vi "Read Wait For Response.vi"(0 "LVx.lvclass in":refnum<class "LVx.lvclass">, 11 "error in (no error)":errorcluster) -> (4 "LVx.lvclass out":refnum<class "LVx.lvclass">, 6 "Wait For Response?":bool, 15 "error out":errorcluster)   [LabVIEW 2011, in "LVx.lvlib" / "LVx.lvclass"]
uses:
  LVx.lvclass
  LVx.lvclass/LVx.ctl
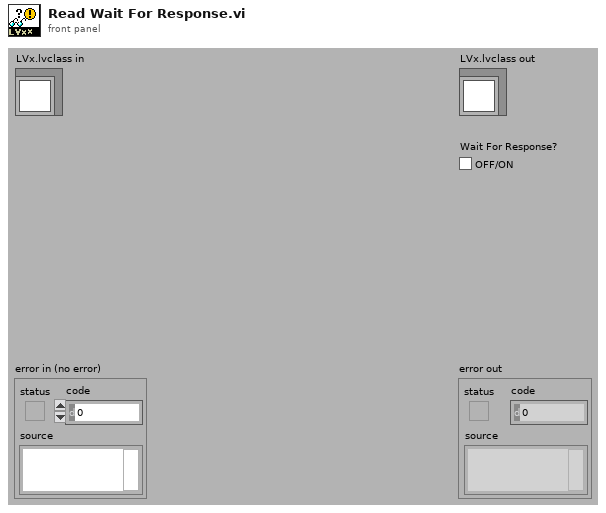
[diagram p1: front panel]
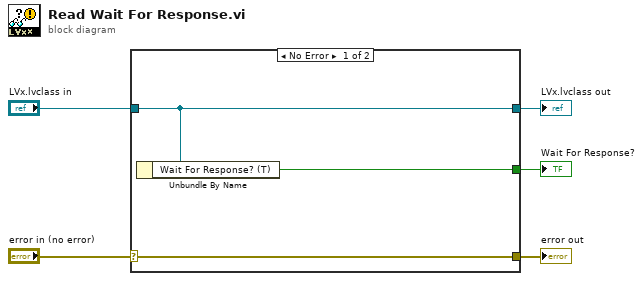
[diagram p0: block diagram]
diagram:
  n1 = case shown="No Error" "error in (no error)" {
    selector: "error in (no error)" -> [w8 w9]
    tunnel: [w8 w9] -> w4
    tunnel: [w7 w10] -> w2
    tunnel: "LVx.lvclass in" -> [w7 w10]
    tunnel: [w6 _] -> w1
    frame No Error {
      n2 = Unbundle By Name(w7) -> ("Wait For Response? (T)"=w6:bool)
    }
    frame Error {
    }
  }
  "error out" <- w4
  "LVx.lvclass out" <- w2
  "Wait For Response?" <- w1
